vi "Autonomous Independent.vi"   [LabVIEW 2019]
doc: "This VI is called when autonomous begins, and will automatically be terminated when autonomous ends. You can carry out timed or sensor driven robot movement independently without needing to return to the caller."
uses:
  Motion_Profiler_Class-master/MotionProfiles.lvclass
  <vilib>/Rock Robotics/WPI/ThirdParty/Phoenix-LabVIEW/Motor Controller/Sensor/CTRE_Phoenix_MotorControl_SetIntegratedSensorPosition_TalonFX.vi
  <vilib>/Rock Robotics/Network Tables/NT Write Variant.vi
  <vilib>/Utility/file.llb/Read Delimited Spreadsheet (string).vi
  <vilib>/Rock Robotics/Network Tables/NT Read String.vi
panel:
  # "Be sure to right-click and choose Data Operations>>Make Current Value default if you want to save the array values with the VI"
types:
  T1 = typedef "WPI_MotorControlDeviceRef.ctl" = cluster{"DeviceStatus":errorcluster, "Type":T2, "PWM":cluster{"PWM Channel":T3, "DeadBand":T4}, "CAN":cluster{"Device Number":u8, "SetOutput VI Ref":variant, "GetOutput VI Ref":variant, "Enable VI Ref":variant, "Disable VI Ref":variant, "Data":variant}, "Invert":bool, "DIO PWM":cluster{"PWM \"Enable\" Channel":T3, "DIOChannel":T5, "PWM Rate":dbl}}
  T2 = typedef "WPI_MotorControlType.ctl" = enum16{"PWM", "CAN", "DIO PWM"}
  T3 = typedef "FPGA_DIOPWMChannel.ctl" = enum8{"PWM 0", "PWM 1", "PWM 2", "PWM 3", "PWM 4", "PWM 5", "PWM 6", "PWM 7", "PWM 8", "PWM 9", "PWM MXP 0", "PWM MXP 1", "PWM MXP 2", "PWM MXP 3", "PWM MXP 4", "PWM MXP 5", "PWM MXP 6", "PWM MXP 7", "PWM MXP 8", "PWM MXP 9", "Invalid"}
  T4 = typedef "WPI_PWMDeadband.ctl" = cluster{"Name":string, "maxPositivePwm":i32, "minPositivePwm":i32, "centerPwm":i32, "maxNegativePwm":i32, "minNegativePwm":i32, "angularRange":u16}
  T5 = typedef "FPGA_DIOChannel.ctl" = enum8{"DIO 0", "DIO 1", "DIO 2", "DIO 3", "DIO 4", "DIO 5", "DIO 6", "DIO 7", "DIO 8", "DIO 9", "DIO MXP 0", "DIO MXP 1", "DIO MXP 2", "DIO MXP 3", "DIO MXP 4", "DIO MXP 5", "DIO MXP 6", "DIO MXP 7", "DIO MXP 8", "DIO MXP 9", "DIO MXP 10", "DIO MXP 11", "DIO MXP 12", "DIO MXP 13", "DIO MXP 14", "DIO MXP 15", "SPI Port CS1", "SPI Port CS2", "SPI Port CS3", "SPI Port MISO", "SPI Port MOSI", "Invalid"}
  T6 = typedef "MotionProfiles.lvclass/MotionProfile_MP_Class_Status.ctl" = cluster{"Motion Profile Status":cluster{"Top Buffer Remaining":i32, "Top Buffer Count":i32, "Bottom Buffer Count":i32, "Has Underrun?":bool, "Is Underrun?":bool, "Active Point Valid?":bool, "Is Last?":bool, "Profile Slot Select 0":i32, "Output Enable":i32, "Time Duration (ms)":i32, "Profile Slot Select 1":i32}, "TalonState":T7, "MP Is Done":bool, "MP Is Executing":bool, "Set_Vel_(u/100ms)":i32, "Set_Pos_(u)":i32, "Act_Vel_(u/100ms)":i32, "Act_Pos(u)":i32, "Throtle":dbl}
  T7 = typedef "MotionProfiles.lvclass/MotionProfile_TalonSetValueEnum.ctl" = enum16{"Disable", "Enable", "Hold"}
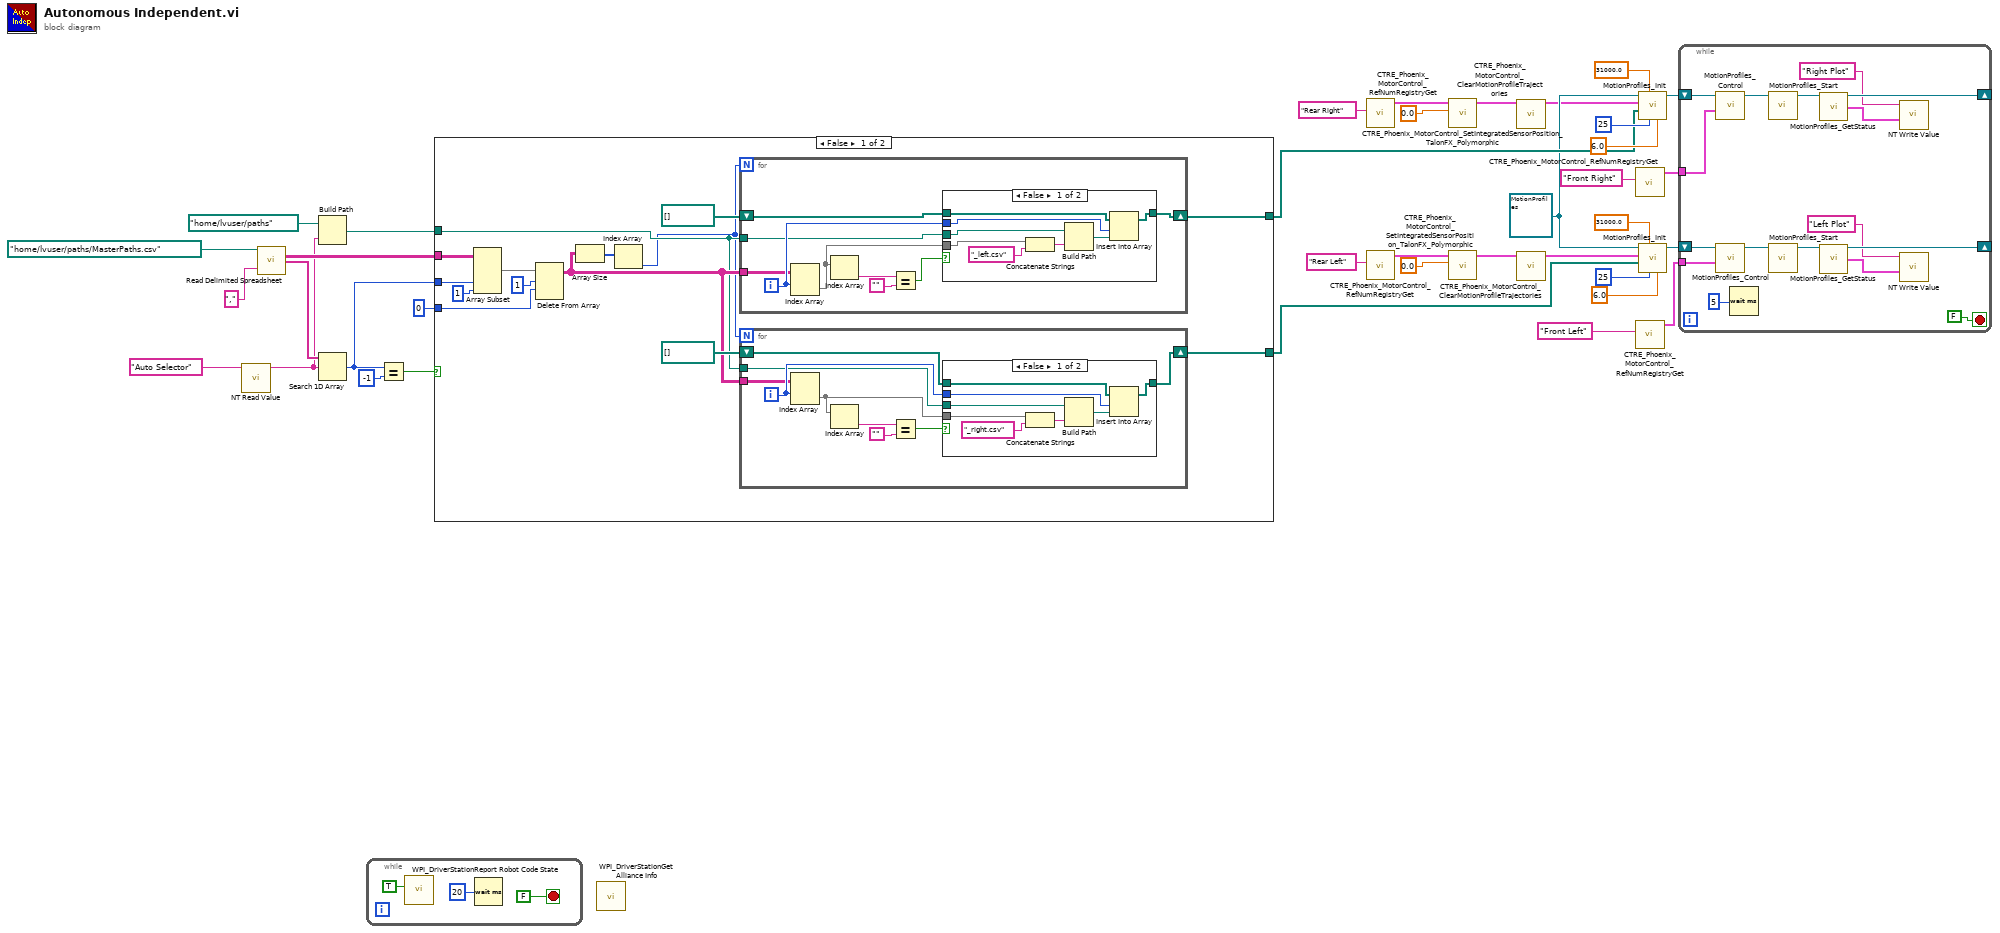
[diagram p0: block diagram]
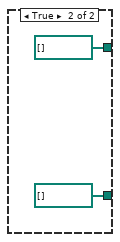
[diagram p4: hidden frame]
diagram:
  w13 = refnum<class "MotionProfiles.lvclass"> refnum ("MotionProfiles.lvclass")
  n1 = call-poly <vilib>:"NT Read Value.vi"("Name"="Auto Selector") -> ("String"=w8:string)  [unwired: 9 in, 1 out]
  n2 = call-poly <vilib>:"Read Delimited Spreadsheet.vi"("file path (dialog if empty)"=path "/home/lvuser/paths/MasterPaths.csv" ("file path (use dialog)"), "delimiter (\\t)"="," ("delimiter (\\t)")) -> ("all rows"=w24:string[][], "first row"=w27:string[])  [unwired: 8 in, 4 out]
  n3 = Build Path(base path=path "/home/lvuser/paths" ("file path (use dialog)"), name or relative path=w8) -> (appended path=w5:path)
  n4 = Search 1D Array(1D array=w27, element=w8) -> (index of element=w23:i32)  [unwired: 1 in]
  n5 = while {
    stop <- FALSE stop-if-true
    n6 = call <vilib>:"WPI_DriverStationReport Robot Code State.vi"("Autonomous"=TRUE) -> ()  [unwired: 10 in, 1 out]
    n7 = Wait (ms)(milliseconds to wait=u32 20) -> ()  [unwired: 1 out]
  }
  n8 = Equal?(x=w23, y=-1) -> (x = y?=w25:bool)
  n9 = case shown="False" w25 {
    tunnel: w24 -> [w54 _]
    tunnel: w23 -> [w46 _]
    tunnel: [w42 path[] [] ("CSV File Path")] -> w18
    tunnel: [w48 path[] [] ("CSV File Path")] -> w14
    tunnel: w5 -> [w43 _]
    tunnel: 0 ("index (row)") -> [w47 _]
    frame False {
      n10 = Array Subset(array=w54, index (col)=w46, length (col)=1 ("length")) -> (w52:string[][])  [unwired: 2 in]
      n11 = Delete From Array(array=w52, length=1, index (row)=w47) -> (array with subset deleted=w44:string[][])  [unwired: 1 in, 1 out]
      n12 = Array Size(array=w44) -> (size(s)=w50:i32[])
      n13 = Index Array(array=w50) -> (element=w41:i32)  [unwired: 1 in]
      n14 = for {
        N: w41 -> [_]
        shift-right: [w62] -> w42
        shift-left: path[] [] ("CSV File Path") -> [w63]
        tunnel: w44 -> [w60]
        tunnel: w43 -> [w55]
        i -> [w61]
        n15 = Index Array(array=w60, index (row)=w61) -> (element=w57:string[])  [unwired: 1 in]
        n16 = Index Array(array=w57) -> (element=w56:string)  [unwired: 1 in]
        n17 = Equal?(x=w56, y="") -> (x = y?=w59:bool)
        n18 = case shown="False" w59 {
          tunnel: w63 -> [w71 w72]
          tunnel: [w70 w72] -> w62
          tunnel: w61 -> [w69 _]
          tunnel: w57 -> [w68 _]
          tunnel: w55 -> [w64 _]
          frame False {
            n19 = Concatenate Strings(w68, "_left.csv" ("string")) -> (w66:string)
            n20 = Build Path(base path=w64, name or relative path=w66) -> (appended path=w65:path)
            n21 = Insert Into Array(array=w71, index=w69, new element=w65) -> (w70:path[])
          }
          frame True {
          }
        }
      }
      n22 = for {
        N: w41 -> [_]
        shift-right: [w80] -> w48
        shift-left: path[] [] ("CSV File Path") -> [w81]
        tunnel: w44 -> [w78]
        tunnel: w43 -> [w77]
        i -> [w79]
        n23 = Index Array(array=w78, index (row)=w79) -> (element=w74:string[])  [unwired: 1 in]
        n24 = Index Array(array=w74) -> (element=w73:string)  [unwired: 1 in]
        n25 = Equal?(x=w73, y="") -> (x = y?=w76:bool)
        n26 = case shown="False" w76 {
          tunnel: w81 -> [w89 w90]
          tunnel: [w88 w90] -> w80
          tunnel: w79 -> [w87 _]
          tunnel: w74 -> [w86 _]
          tunnel: w77 -> [w82 _]
          frame False {
            n27 = Concatenate Strings(w86, "_right.csv" ("string")) -> (w84:string)
            n28 = Build Path(base path=w82, name or relative path=w84) -> (appended path=w83:path)
            n29 = Insert Into Array(array=w89, index=w87, new element=w83) -> (w88:path[])
          }
          frame True {
          }
        }
      }
    }
    frame True {
    }
  }
  n30 = call <vilib>:"WPI_DriverStationGet Alliance Info.vi"() -> ()  [unwired: 12 out]
  n31 = call <vilib>:"CTRE_Phoenix_MotorControl_RefNumRegistryGet.vi"("refnum name"="Rear Right") -> ("PhoenixMotorControlDevRef"=w30:T1)  [unwired: 9 in, 1 out]
  n32 = call <vilib>:"CTRE_Phoenix_MotorControl_RefNumRegistryGet.vi"("refnum name"="Rear Left") -> ("PhoenixMotorControlDevRef"=w32:T1)  [unwired: 9 in, 1 out]
  n33 = call-poly <vilib>:"CTRE_Phoenix_MotorControl_SetIntegratedSensorPosition_TalonFX_Polymorphic.vi"("New Position"=0.0, "PhoenixMotorControlDevRef"=w30) -> ("PhoenixMotorControlDevRef"=w4:T1)  [unwired: 8 in, 1 out]
  n34 = call-poly <vilib>:"CTRE_Phoenix_MotorControl_SetIntegratedSensorPosition_TalonFX_Polymorphic.vi"("New Position"=0.0, "PhoenixMotorControlDevRef"=w32) -> ("PhoenixMotorControlDevRef"=w2:T1)  [unwired: 8 in, 1 out]
  n35 = call <vilib>:"CTRE_Phoenix_MotorControl_ClearMotionProfileTrajectories.vi"("PhoenixMotorControlDevRef"=w4) -> ("PhoenixMotorControlDevRef"=w3:T1)  [unwired: 13 in, 1 out]
  n36 = call <vilib>:"CTRE_Phoenix_MotorControl_ClearMotionProfileTrajectories.vi"("PhoenixMotorControlDevRef"=w2) -> ("PhoenixMotorControlDevRef"=w1:T1)  [unwired: 13 in, 1 out]
  n37 = call <vilib>:"CTRE_Phoenix_MotorControl_RefNumRegistryGet.vi"("refnum name"="Front Right") -> ("PhoenixMotorControlDevRef"=w9:T1)  [unwired: 9 in, 1 out]
  n38 = call <vilib>:"CTRE_Phoenix_MotorControl_RefNumRegistryGet.vi"("refnum name"="Front Left") -> ("PhoenixMotorControlDevRef"=w10:T1)  [unwired: 9 in, 1 out]
  n39 = call "MotionProfiles_Init.vi"("Wheel_Diameter (in)"=6.0, "MP_Frame_Rate_(ms)"=25, "Encoder_CPR_4x"=31000.0, "CSV File Path"=w18, "PhoenixMotorControlDevRef"=w3, "MotionProfiles in"=w13) -> ("MotionProfiles out"=w12:refnum<class "MotionProfiles.lvclass">)  [unwired: 4 in, 1 out]
  n40 = call "MotionProfiles_Init.vi"("Wheel_Diameter (in)"=6.0, "MP_Frame_Rate_(ms)"=25, "Encoder_CPR_4x"=31000.0, "CSV File Path"=w14, "PhoenixMotorControlDevRef"=w1, "MotionProfiles in"=w13) -> ("MotionProfiles out"=w11:refnum<class "MotionProfiles.lvclass">)  [unwired: 4 in, 1 out]
  n41 = while {
    shift-right: [w97] -> _
    shift-left: w12 -> [w104]
    shift-right: [w98] -> _
    shift-left: w11 -> [w103]
    tunnel: w10 -> [w102]
    tunnel: w9 -> [w101]
    stop <- FALSE stop-if-true
    n42 = call "MotionProfiles_Control.vi"("PhoenixMotorControlDevRef Slave"=w101, "MotionProfiles in"=w104) -> ("MotionProfiles out"=w106:refnum<class "MotionProfiles.lvclass">)  [unwired: 8 in, 1 out]
    n43 = call "MotionProfiles_Control.vi"("PhoenixMotorControlDevRef Slave"=w102, "MotionProfiles in"=w103) -> ("MotionProfiles out"=w105:refnum<class "MotionProfiles.lvclass">)  [unwired: 8 in, 1 out]
    n44 = Wait (ms)(milliseconds to wait=u32 5) -> ()  [unwired: 1 out]
    n45 = call "MotionProfiles_Start.vi"("MotionProfiles in"=w106) -> ("MotionProfiles out"=w100:refnum<class "MotionProfiles.lvclass">)  [unwired: 9 in, 1 out]
    n46 = call "MotionProfiles_Start.vi"("MotionProfiles in"=w105) -> ("MotionProfiles out"=w99:refnum<class "MotionProfiles.lvclass">)  [unwired: 9 in, 1 out]
    n47 = call "MotionProfiles_GetStatus.vi"("MotionProfiles in"=w100) -> ("MotionProfiles out"=w97:refnum<class "MotionProfiles.lvclass">, "MP_Class_Status"=w96:T6)  [unwired: 12 in, 1 out]
    n48 = call "MotionProfiles_GetStatus.vi"("MotionProfiles in"=w99) -> ("MotionProfiles out"=w98:refnum<class "MotionProfiles.lvclass">, "MP_Class_Status"=w93:T6)  [unwired: 12 in, 1 out]
    n49 = call-poly <vilib>:"NT Write Value.vi"("Variant"=w96, "Name"="Right Plot") -> ()  [unwired: 9 in, 1 out]
    n50 = call-poly <vilib>:"NT Write Value.vi"("Variant"=w93, "Name"="Left Plot") -> ()  [unwired: 9 in, 1 out]
  }
